vi "static.vi"(8 "error in (no error)":errorcluster, 11 "parent in":refnum<class "Parent.lvclass">) -> (0 "error out":errorcluster, 2 "message":string="Parent Static  VI", 3 "parent out":refnum<class "Parent.lvclass">)   [LabVIEW 2024, in "Parent.lvclass"]
uses:
  Parent.lvclass
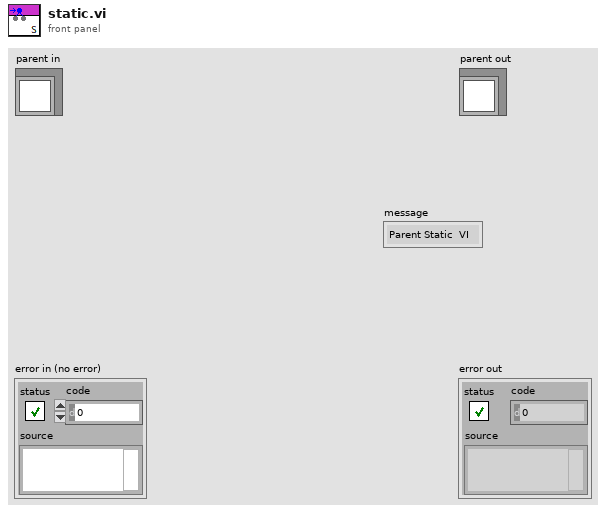
[diagram p1: front panel]
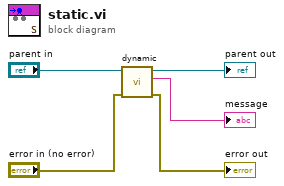
[diagram p0: block diagram]
diagram:
  n1 = call-dynamic "dynamic.vi"("error in (no error)"="error in (no error)", "parent in"="parent in") -> ("error out"=→"error out":errorcluster, "message"=→"message":string, "parent out"=→"parent out":refnum<class "Parent.lvclass">)  [unwired: 7 in]
